vi "Pid_v11.vi"() -> ()   [LabVIEW 2020]
panel:
  out "u - Comanda":dbl(graph)=48.656716417098906
  out "y - Iesirea":dbl(slide)=48.65671641792066 scale=40.0..60.0
  in  "stop":bool
  out "y":dbl=48.65671641792066
  out "u":dbl(slide)=48.65671641709671 scale=40.0..60.0
  out "u,y,r":cluster{"r-Set point":dbl, dbl, dbl}(graph)={"r-Set point"=48.656716417910445, 48.65671641792066, 48.656716417098906}
  in  "Kd":dbl(slide)=0.1111111111111111 scale=0.0..0.5
  in  "Kp":dbl(slide)=0.3508771929824561 scale=0.0..2.5
  in  "Ki":dbl(slide)=0.8888888888888888 scale=0.0..2.0
  in  "r-Set point":dbl(slide)=48.656716417910445 scale=40.0..60.0
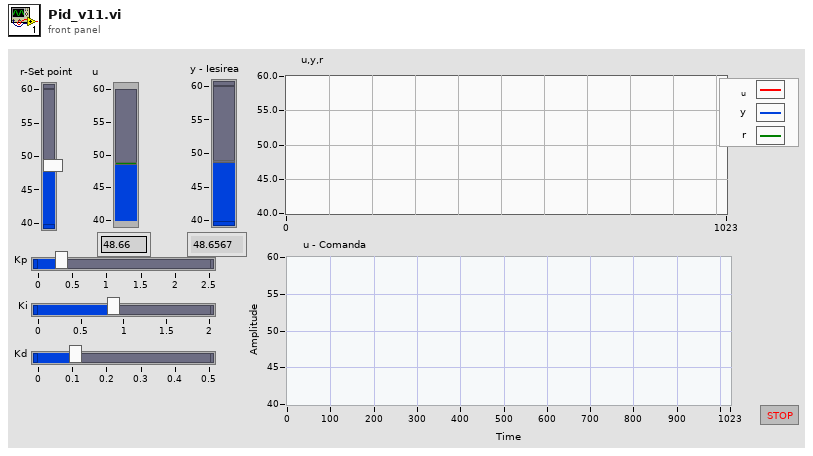
[diagram p1: front panel]
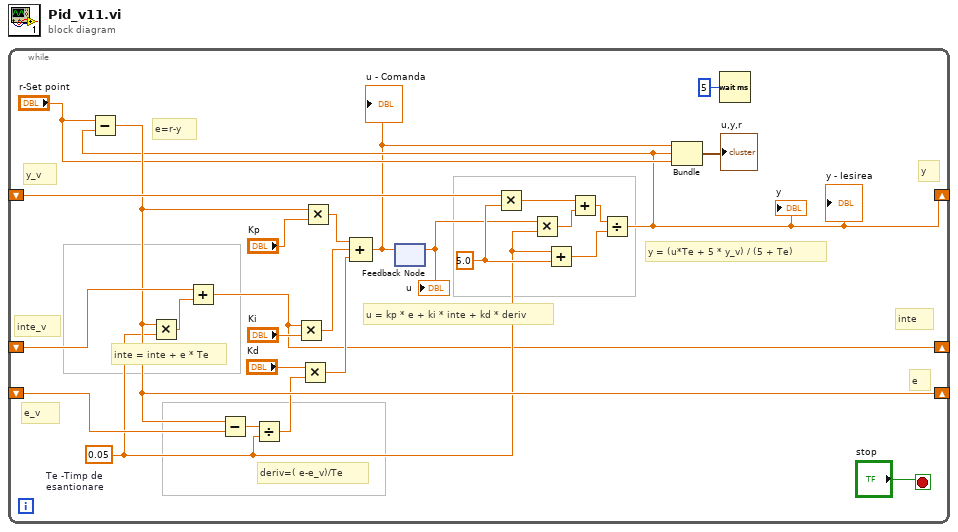
[diagram p0: block diagram]
diagram:
  n1 = while {
    shift-right: [w17] -> _
    shift-left: _ -> [w16]
    shift-right: [w3] -> _
    shift-left: _ -> [w18]
    shift-right: [w5] -> _
    shift-left: _ -> [w20]
    stop <- "stop" stop-if-true
    w22 = 5.0 ("y")
    w7 = 0.05  # Te -Timp de  esantionare
    # "u = kp * e + ki * inte + kd * deriv"
    # "e_v"
    # "e"
    # "inte_v"
    # "inte"
    # "y_v"
    # "y"
    # "inte = inte + e * Te"
    # "e=r-y"
    # "deriv=( e-e_v)/Te"
    # "y = (u*Te + 5 * y_v) / (5 + Te)"
    n2 = feedback #1() -> (w13:dbl)  [unwired: 1 in]
    "u" <- w13
    n3 = Multiply(x=w18, y=w22) -> (x*y=w24:dbl)
    n4 = Multiply(x=w13, y=w7) -> (x*y=w25:dbl)
    n5 = Add(x=w7, y=w22) -> (x+y=w23:dbl)
    n6 = Add(x=w24, y=w25) -> (x+y=w26:dbl)
    n7 = Divide(x=w26, y=w23) -> (x/y=w3:dbl)
    "y" <- w3
    "y - Iesirea" <- w3
    n8 = Subtract(x="r-Set point", y=w3) -> (x-y=w17:dbl)
    n9 = Multiply(x=w17, y=w7) -> (x*y=w6:dbl)
    n10 = Add(x=w20, y=w6) -> (x+y=w5:dbl)
    n11 = Subtract(x=w17, y=w16) -> (x-y=w15:dbl)
    n12 = Divide(x=w15, y=w7) -> (x/y=w11:dbl)
    n13 = Multiply(x=w5, y="Ki") -> (x*y=w9:dbl)
    n14 = Multiply(x="Kd", y=w11) -> (x*y=w8:dbl)
    n15 = Multiply(x=w17, y="Kp") -> (x*y=w10:dbl)
    n16 = Compound Arithmetic op=ADD(w10, w9, w8) -> (w2:dbl)
    "u - Comanda" <- w2
    n17 = feedback-in #1(w2) -> ()
    n18 = Bundle(w2, w3, "r-Set point"="r-Set point") -> (→"u,y,r":cluster{dbl, dbl, "r-Set point":dbl})  [unwired: 1 in]
    n19 = Wait (ms)(milliseconds to wait=u32 5) -> ()  [unwired: 1 out]
  }
